vi "RTP_RTSP - Parse H264 NAL units.vi"(5 "H264 NAL unit":T1, 7 "New Payload":string) -> (6 "H264 NAL unit 2":T1)   [LabVIEW 2014]
uses:
  H264 NAL unit.ctl
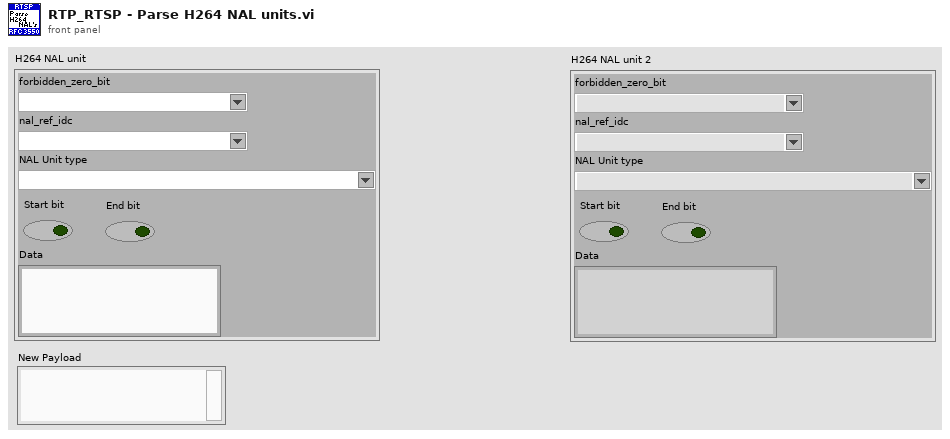
[diagram p1: front panel]
types:
  T1 = typedef "H264 NAL unit.ctl" = cluster{"forbidden_zero_bit":string, "nal_ref_idc":string, "NAL Unit type":string, "Start bit":bool, "End bit":bool, "Data":string}
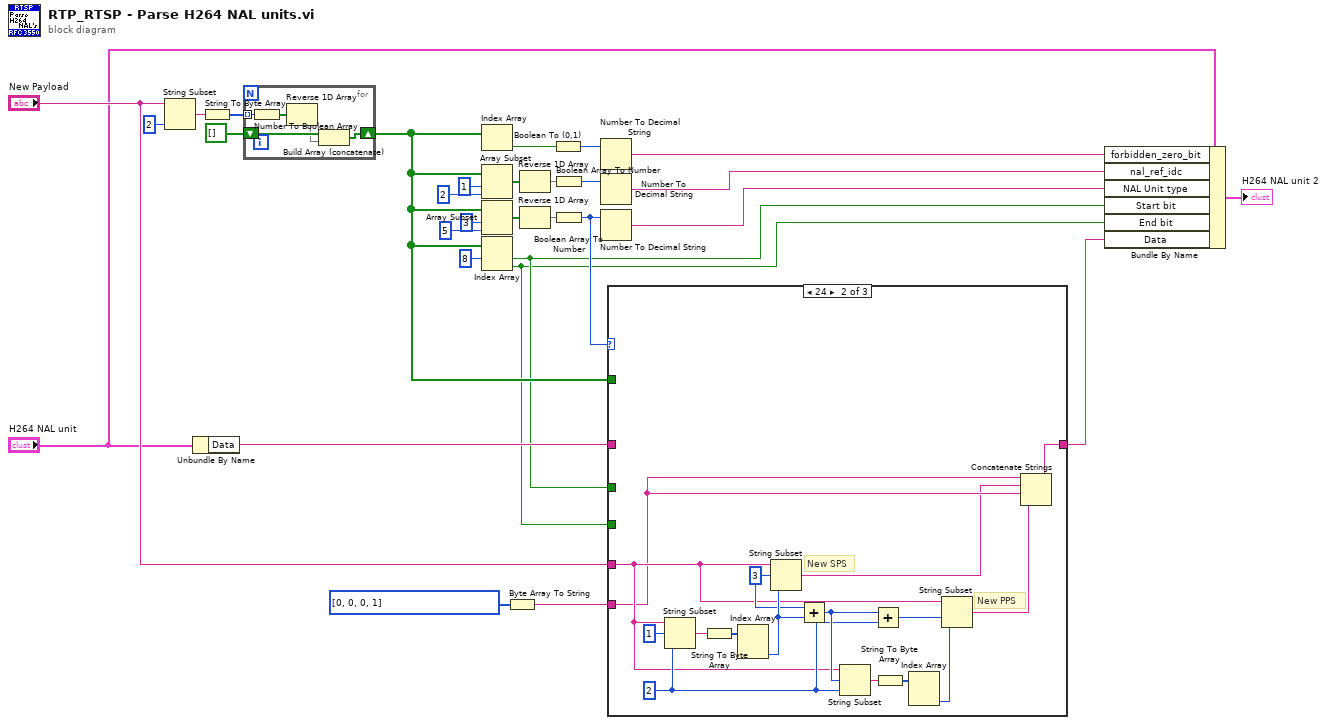
[diagram p0: block diagram]
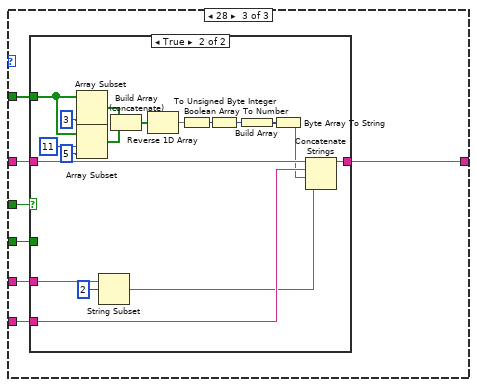
[diagram p3: hidden frame]
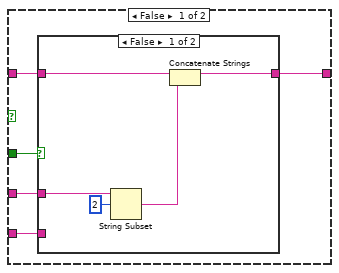
[diagram p4: hidden frame]
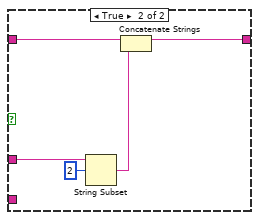
[diagram p5: hidden frame]
diagram:
  n1 = String Subset(string="New Payload", length (rest)=2 ("length (rest)")) -> (substring=w18:string)  [unwired: 1 in]
  n2 = Unbundle By Name("H264 NAL unit") -> ("Data"=w8:string)
  n3 = String To Byte Array(string=w18) -> (unsigned byte array=w29:u8[])
  n4 = for {
    tunnel: w29 -> [w35] mode=indexing
    shift-right: [w32] -> w10
    shift-left: bool[] [] -> [w34]
    n5 = Number To Boolean Array(number=w35) -> (Boolean array=w33:bool[])
    n6 = Reverse 1D Array(array=w33) -> (reversed array=w31:bool[])
    n7 = Build Array (concatenate)(w34, w31) -> (w32:bool[])
  }
  n8 = Index Array(array=w10) -> (element=w28:bool)  [unwired: 1 in]
  n9 = Array Subset(array=w10, index=1, length=2) -> (w11:bool[])
  n10 = Array Subset(array=w10, index=3, length=5) -> (w12:bool[])
  n11 = Index Array(array=w10, index #1=8 ("index")) -> (element #1=w2:bool, element #2=w1:bool)  [unwired: 1 in]
  n12 = Byte Array To String(unsigned byte array=u8[] [0, 0, 0, 1]) -> (string=w13:string)
  n13 = Reverse 1D Array(array=w11) -> (reversed array=w25:bool[])
  n14 = Reverse 1D Array(array=w12) -> (reversed array=w20:bool[])
  n15 = Boolean To (0,1)(Boolean=w28) -> (0, 1=w27:i16)
  n16 = Boolean Array To Number(Boolean array=w25) -> (number=w26:u32)
  n17 = Boolean Array To Number(Boolean array=w20) -> (number=w16:u32)
  n18 = Number To Decimal String(number=w27) -> (decimal integer string=w5:string)  [unwired: 1 in]
  n19 = Number To Decimal String(number=w26) -> (decimal integer string=w4:string)  [unwired: 1 in]
  n20 = Number To Decimal String(number=w16) -> (decimal integer string=w3:string)  [unwired: 1 in]
  n21 = case shown="24" w16 {
    tunnel: "New Payload" -> [_ w42 w58]
    tunnel: w2 -> [_ _ w59]
    tunnel: w1 -> [_ _ w57]
    tunnel: w13 -> [_ w40 w56]
    tunnel: w10 -> [_ _ w55]
    tunnel: w8 -> [w36 _ w54]
    tunnel: [w36 w37 w53] -> w7
    frame 0, Default {
    }
    frame 24 {
      w43 = 2 ("length (rest)")
      w49 = 3 ("length (rest)")
      # "New PPS"
      # "New SPS"
      n22 = String Subset(string=w42, offset (0)=1, length (rest)=w43) -> (substring=w52:string)
      n23 = String To Byte Array(string=w52) -> (unsigned byte array=w51:u8[])
      n24 = Index Array(array=w51) -> (element #2=w50:u8)  [unwired: 2 in, 1 out]
      n25 = String Subset(string=w42, offset (0)=w49, length (rest)=w50) -> (substring=w39:string)
      n26 = Add(x=w49, y=w50) -> (x+y=w44:i32)
      n27 = String Subset(string=w42, offset (0)=w44, length (rest)=w43) -> (substring=w46:string)
      n28 = Add(x=w44, y=w43) -> (x+y=w41:i32)
      n29 = String To Byte Array(string=w46) -> (unsigned byte array=w47:u8[])
      n30 = Index Array(array=w47) -> (element #2=w45:u8)  [unwired: 2 in, 1 out]
      n31 = String Subset(string=w42, offset (0)=w41, length (rest)=w45) -> (substring=w38:string)
      n32 = Concatenate Strings(w40, w39, w40, w38) -> (w37:string)
    }
    frame 28 {
      n33 = case shown="True" w59 {
        tunnel: w54 -> [w63 w79]
        tunnel: w58 -> [w62 w91]
        tunnel: w57 -> [w64 _]
        tunnel: w56 -> [w61 w78]
        tunnel: w55 -> [_ w88]
        tunnel: [w60 w75] -> w53
        frame False {
          n34 = case shown="False" w64 {
            tunnel: w63 -> [w67 w72]
            tunnel: w62 -> [w68 w73]
            tunnel: w61 -> [_ _]
            tunnel: [w65 w70] -> w60
            frame False {
              n35 = String Subset(string=w68, offset (0)=2 ("length (rest)")) -> (substring=w66:string)  [unwired: 1 in]
              n36 = Concatenate Strings(w67, w66) -> (w65:string)
            }
            frame True {
              n37 = String Subset(string=w73, offset (0)=2 ("length (rest)")) -> (substring=w71:string)  [unwired: 1 in]
              n38 = Concatenate Strings(w72, w71) -> (w70:string)
            }
          }
        }
        frame True {
          n39 = Array Subset(array=w88, length=3) -> (w86:bool[])  [unwired: 1 in]
          n40 = Array Subset(array=w88, index=11, length=5) -> (w85:bool[])
          n41 = String Subset(string=w91, offset (0)=2) -> (substring=w76:string)  [unwired: 1 in]
          n42 = Build Array (concatenate)(w86, w85) -> (w80:bool[])
          n43 = Reverse 1D Array(array=w80) -> (reversed array=w81:bool[])
          n44 = Boolean Array To Number(Boolean array=w81) -> (number=w84:u32)
          n45 = To Unsigned Byte Integer(number=w84) -> (unsigned 8bit integer=w82:u8)
          n46 = Build Array(w82) -> (w83:u8[])
          n47 = Byte Array To String(unsigned byte array=w83) -> (string=w77:string)
          n48 = Concatenate Strings(w79, w78, w77, w76) -> (w75:string)
        }
      }
    }
  }
  n49 = Bundle By Name(cluster="H264 NAL unit", "forbidden_zero_bit"=w5, "nal_ref_idc"=w4, "NAL Unit type"=w3, "Start bit"=w2, "End bit"=w1, "Data"=w7) -> (→"H264 NAL unit 2":T1)
